vi "Bookmark整体图.vi"() -> ()   [LabVIEW 2014]
panel:
  in  "Amor":bool
  in  "Toolbar":bool
  in  "List":bool
  in  "Folder":bool
  in  "Favorite":bool
  in  "Edit":bool
  in  "Create":bool
  in  "Bookmark":bool
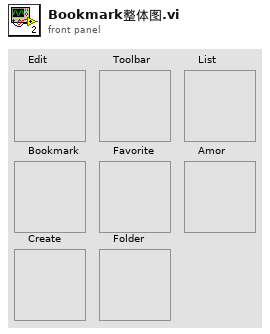
[diagram p1: front panel]
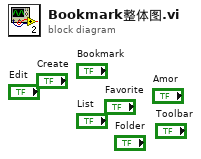
[diagram p0: block diagram]
diagram:
